vi "setStages.vi"(8 "error in (no error)":errorcluster, 10 "Stage":T1(ring), 11 "RfRamp.lvclass in":refnum<class "RfRamp.lvclass">) -> (0 "error out":errorcluster, 3 "RfRamp.lvclass out":refnum<class "RfRamp.lvclass">)   [LabVIEW 2009, in "Tools.lvlib" / "Scripting.lvlib" / "RfRamp.lvclass"]
uses:
  RfRamp.lvclass
  Rf Event/rf.lvclass
  RfRamp.lvclass/RfRamp.ctl
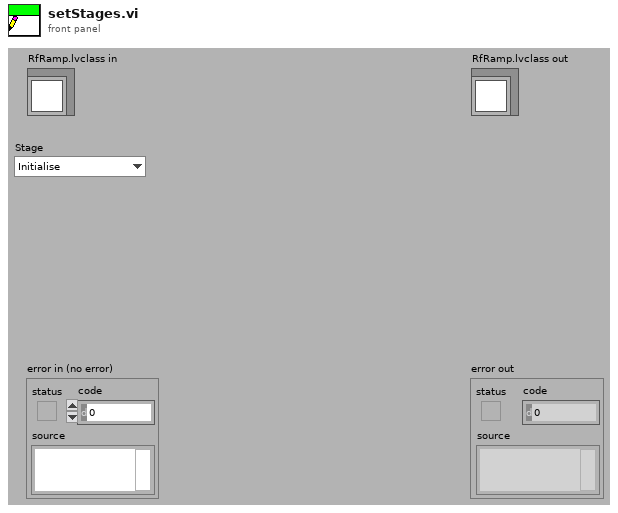
[diagram p1: front panel]
types:
  T1 = enum16{"Initialise", "MOT", "Molasses", "Optical Pumping", "Magnetic Trap", "RF Cooling", "Manipulation", "Switch Off", "Absorption Imaging", "Fluorscence Imaging", "Shut Down"}
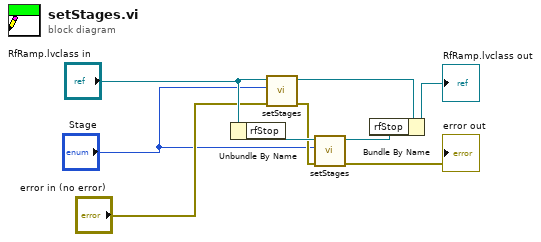
[diagram p0: block diagram]
diagram:
  n1 = Unbundle By Name("RfRamp.lvclass in") -> ("rfStop"=w9:refnum<class "rf.lvclass">)
  n2 = call-parent "setStages.vi"("error in (no error)"="error in (no error)", "Stage"="Stage", "ScriptEvent.lvclass in"="RfRamp.lvclass in") -> ("error out"=w6:errorcluster, "ScriptEvent.lvclass out"=w8:refnum<class "RfRamp.lvclass">)  [unwired: 7 in]
  n3 = call-parent "setStages.vi"("error in (no error)"=w6, "Stage"="Stage", "ScriptEvent.lvclass in"=w9) -> ("error out"=→"error out":errorcluster, "ScriptEvent.lvclass out"=w7:refnum<class "rf.lvclass">)  [unwired: 7 in]
  n4 = Bundle By Name(cluster=w8, "rfStop"=w7) -> (→"RfRamp.lvclass out":refnum<class "RfRamp.lvclass">)
